vi "X,Y,Z轴坐标查询NEW.vi"(2 "细分设置":dbl, 3 "查询坐标轴":string, 4 "串口通信端口":refnum<visa-resource-name>) -> (0 "坐标(mm)":dbl, 1 "VISA O":refnum<visa-resource-name>)   [LabVIEW 2016]
panel:
  # "XYZ轴坐标查询"
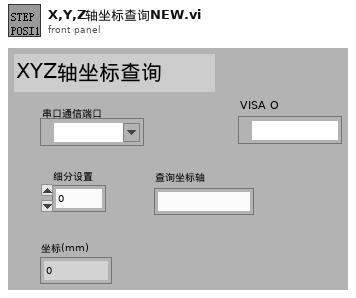
[diagram p1: front panel]
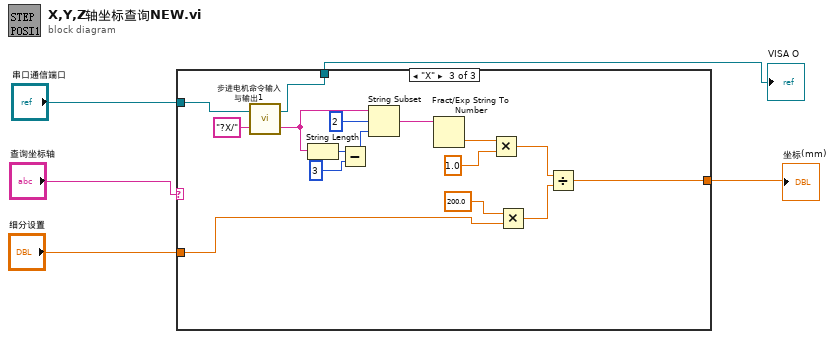
[diagram p0: block diagram]
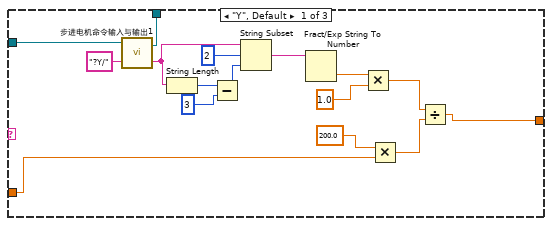
[diagram p2: hidden frame]
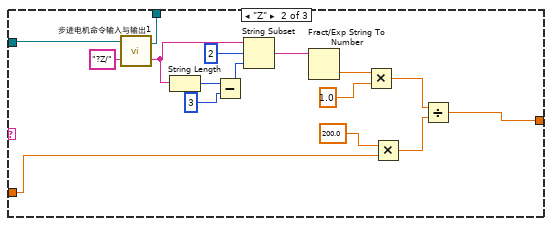
[diagram p3: hidden frame]
diagram:
  n1 = case shown="\"X\"" "查询坐标轴" {
    tunnel: "串口通信端口" -> [w9 w26 w41]
    tunnel: "细分设置" -> [w8 w25 w40]
    tunnel: [w7 w23 w39] -> w2
    tunnel: [w6 w22 w38] -> w1
    frame "Y", Default {
      n2 = call "步进电机命令输入与输出1.vi"("输入字符串"="?Y/", "串口通信端口"=w9) -> ("返回字符串"=w14:string, "VISA资源名称输出"=w6:refnum<visa-resource-name>)
      n3 = String Length(string=w14) -> (length=w12:i32)
      n4 = Subtract(x=w12, y=3) -> (x-y=w15:i32)
      n5 = String Subset(string=w14, offset (0)=2 ("偏移量(0)"), length (rest)=w15) -> (substring=w16:string)
      n6 = Fract/Exp String To Number(string=w16) -> (number=w17:dbl)  [unwired: 4 out]
      n7 = Multiply(x=w17, y=1.0) -> (x*y=w21:dbl)
      n8 = Multiply(x=200.0, y=w8) -> (x*y=w20:dbl)
      n9 = Divide(x=w21, y=w20) -> (x/y=w7:dbl)
    }
    frame "Z" {
      n10 = call "步进电机命令输入与输出1.vi"("输入字符串"="?Z/", "串口通信端口"=w26) -> ("返回字符串"=w31:string, "VISA资源名称输出"=w22:refnum<visa-resource-name>)
      n11 = String Length(string=w31) -> (length=w29:i32)
      n12 = Subtract(x=w29, y=3) -> (x-y=w32:i32)
      n13 = String Subset(string=w31, offset (0)=2 ("偏移量(0)"), length (rest)=w32) -> (substring=w33:string)
      n14 = Fract/Exp String To Number(string=w33) -> (number=w34:dbl)  [unwired: 4 out]
      n15 = Multiply(x=w34, y=1.0) -> (x*y=w37:dbl)
      n16 = Multiply(x=200.0, y=w25) -> (x*y=w24:dbl)
      n17 = Divide(x=w37, y=w24) -> (x/y=w23:dbl)
    }
    frame "X" {
      n18 = call "步进电机命令输入与输出1.vi"("输入字符串"="?X/", "串口通信端口"=w41) -> ("返回字符串"=w49:string, "VISA资源名称输出"=w38:refnum<visa-resource-name>)
      n19 = String Length(string=w49) -> (length=w51:i32)
      n20 = Subtract(x=w51, y=3) -> (x-y=w48:i32)
      n21 = String Subset(string=w49, offset (0)=2 ("偏移量(0)"), length (rest)=w48) -> (substring=w47:string)
      n22 = Fract/Exp String To Number(string=w47) -> (number=w46:dbl)  [unwired: 4 out]
      n23 = Multiply(x=w46, y=1.0) -> (x*y=w42:dbl)
      n24 = Multiply(x=200.0, y=w40) -> (x*y=w43:dbl)
      n25 = Divide(x=w42, y=w43) -> (x/y=w39:dbl)
    }
  }
  "坐标(mm)" <- w2
  "VISA O" <- w1
